vi "DMA H-T FIFO Read U32.vi"(0 "Ready for Output?":bool, 1 "FIFO In":refnum<k21>="TX") -> (4 "Data Out":u32, 6 "Data Valid?":bool)   [LabVIEW 2012]
doc: "FIFO Read\n\nThis VI is intended to be used as a wrapper around FIFOs. 4 Wire handshaking has been added."
uses:
  <vilib>/rvi/DataTransferAndStorage/Container/Common/niFpgaContainerExecOnDevCompGetState.vi
  <vilib>/rvi/Emulation/niFpgaSctlEmulationGetInTimedLoop.vi
  <vilib>/rvi/DataTransferAndStorage/Container/Common/niFpgaContainerGetUniqueNameForEmu.vi
  <vilib>/rvi/FIFO/Fifo_Resource/nirvififoEmulationSetSize.vi
  <vilib>/rvi/Emulation/niFpgaSctlEmulationFifoFullMgr.vi
  <vilib>/rvi/errors/niFpgaSetErrorForExecOnDevCompSimple.vi
  <vilib>/rvi/eio/common/nirviEmuReportErrorAndStop.vi
  <vilib>/rvi/interface/RandomDataEmulation/nirviRandomDataFPGAFIFO.vi
  <vilib>/rvi/interface/RandomDataEmulation/niFpgaRandomDataHandleErrors.vi
  <vilib>/rvi/DataTransferAndStorage/Container/XNode/niFpgaContainer.xnode
  <vilib>/rvi/FIFO/Fifo_Resource/niFpgaFifoEmulationRefIn.vi
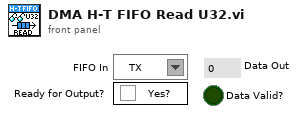
[diagram p1: front panel]
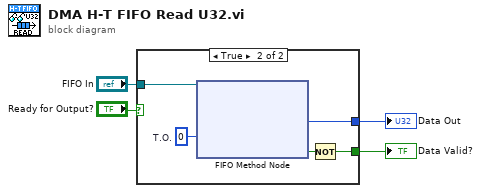
[diagram p0: block diagram]
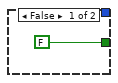
[diagram p2: hidden frame]
diagram:
  n1 = case shown="True" "Ready for Output?" {
    tunnel: [FALSE w10] -> w4
    tunnel: [_ w8] -> w3
    tunnel: "FIFO In" -> [_ w6]
    frame False {
    }
    frame True {
      w7 = 0  # T.O.
      # "Place FIFO Here"
      n2 = xnode ("FIFO Method Node")("Timeout"=w7, "FIFO In"=w6) -> ("Element"=w8:u32, "Timed Out?"=w9:bool)  [unwired: 1 out]
      n3 = Not(x=w9) -> (.not. x?=w10:bool)
    }
  }
  "Data Valid?" <- w4
  "Data Out" <- w3
